vi "fgv_gnss_nmea-data.vi"(7 "cmd":T5, 11 "nmea-data":T4={"$GPGGA-message_OUT"={"TimeStamp"=timestamp(0 s since 1904-01-01), "Latitude"=0.0, "Latitude-Direction"=enum."", "Longitude"=1.0, "Longitude-Direction"=enum."", "GPS-Quality"=enum."GPS fix (SPS)", "N of Satellites"=0, "HDOP"=0.0, "Altitude above Mean-Sea-Level"=0.0, "Geoidal separation"=0.0, "Time since last DGPS update"=0.0, "DGPS reference station ID"=0}} {"$GPGGA-message_OUT"."Time since last DGPS update" format="%.02f [s]"; "$GPGGA-message_OUT"."Geoidal separation" format="%.02f [m]"; "$GPGGA-message_OUT"."Altitude above Mean-Sea-Level" format="%.02f [m]"; "$GPGGA-message_OUT"."HDOP" format="%.02f [HDOP]"; "$GPGGA-message_OUT"."Longitude" format="%0.4f [long]"; "$GPGGA-message_OUT"."Latitude" format="%.04f [lat]"; "$GPGGA-message_OUT"."TimeStamp" format="%<%.2X>T"}) -> (3 "nmea-data out":T4={"$GPGGA-message_OUT"={"TimeStamp"=timestamp(0 s since 1904-01-01), "Latitude"=0.0, "Latitude-Direction"=enum."", "Longitude"=1.0, "Longitude-Direction"=enum."", "GPS-Quality"=enum."GPS fix (SPS)", "N of Satellites"=0, "HDOP"=0.0, "Altitude above Mean-Sea-Level"=0.0, "Geoidal separation"=0.0, "Time since last DGPS update"=0.0, "DGPS reference station ID"=0}} {"$GPGGA-message_OUT"."Time since last DGPS update" format="%.02f [s]"; "$GPGGA-message_OUT"."Geoidal separation" format="%.02f [m]"; "$GPGGA-message_OUT"."Altitude above Mean-Sea-Level" format="%.02f [m]"; "$GPGGA-message_OUT"."HDOP" format="%.02f [HDOP]"; "$GPGGA-message_OUT"."Longitude" format="%0.4f [long]"; "$GPGGA-message_OUT"."Latitude" format="%.04f [lat]"; "$GPGGA-message_OUT"."TimeStamp" format="%<%.2X>T"})   [LabVIEW 2019]
uses:
  Ctrl/cmd_common.ctl
  NMEA_v1.1/NMEA_LatitudeDirection.ctl
  NMEA_v1.1/NMEA_LongitudeDirection.ctl
  NMEA_v1.1/NMEA_GPS-Quality.ctl
  NMEA_v1.1/NMEA.lvlib
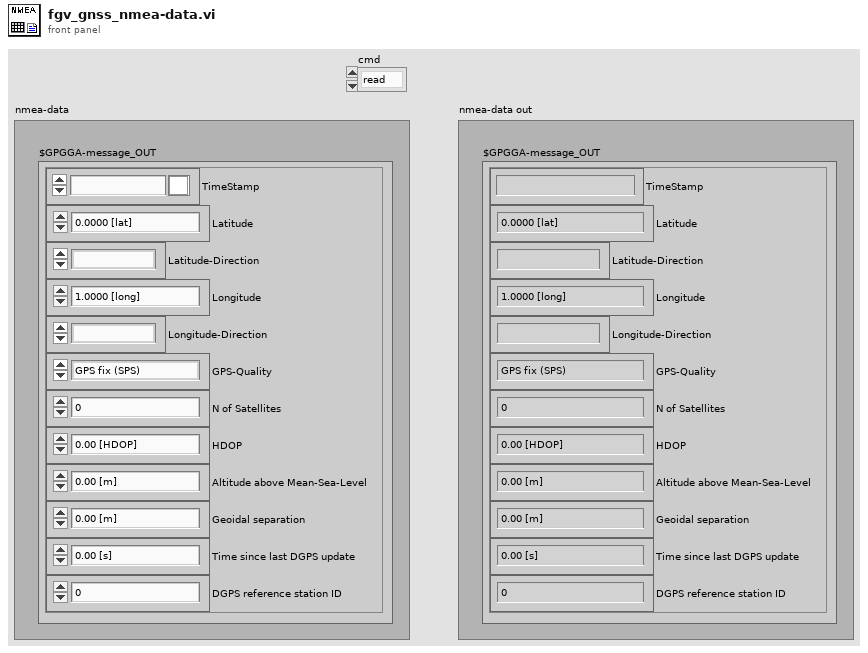
[diagram p1: front panel]
types:
  T1 = typedef "NMEA.lvlib/NMEA_LatitudeDirection.ctl" = enum16{"", "North", "South"}
  T2 = typedef "NMEA.lvlib/NMEA_LongitudeDirection.ctl" = enum16{"", "East", "West"}
  T3 = typedef "NMEA.lvlib/NMEA_GPS-Quality.ctl" = enum16{"Invalid", "GPS fix (SPS)", "DGPS fix", "PPS fix", "Real Time Kinematic", "Float RTK", "estimated", "Manual input mode", "Simulation mode"}
  T4 = cluster{"$GPGGA-message_OUT":cluster{"TimeStamp":timestamp, "Latitude":dbl, "Latitude-Direction":T1, "Longitude":dbl, "Longitude-Direction":T2, "GPS-Quality":T3, "N of Satellites":i32, "HDOP":dbl, "Altitude above Mean-Sea-Level":dbl, "Geoidal separation":dbl, "Time since last DGPS update":dbl, "DGPS reference station ID":i32}}
  T5 = typedef "cmd_common.ctl" = enum16{"read", "write"}
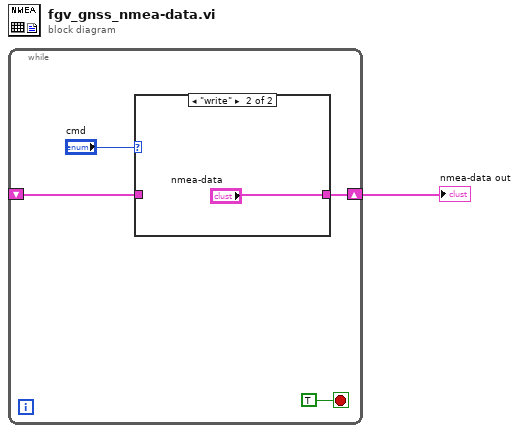
[diagram p0: block diagram]
diagram:
  n1 = while {
    shift-right: [w3] -> w1
    shift-left: _ -> [w2]
    stop <- TRUE stop-if-true
    n2 = case shown="\"write\"" "cmd" {
      tunnel: [w6 "nmea-data"] -> w3
      tunnel: w2 -> [w6 _]
      frame "read", Default {
      }
      frame "write" {
      }
    }
  }
  "nmea-data out" <- w1
